vi "add_line_shifted_enface_IMAQ.vi"(0 "En Face Image":T1, 1 "Shift":dbl=1.0, 5 "Raw Image":T1, 7 "Aspect Ratio":dbl=1.0, 9 "Input Line":dbl=1.0, 11 "error in (no error)":errorcluster, 12 "Output Line":i32) -> (4 "En Face Image Out":T1, 15 "error out":errorcluster)   [LabVIEW 2016]
uses:
  <vilib>/vision/Image Controls.llb/IMAQ Image.ctl
  <vilib>/vision/NI_Vision_Development_Module.lvlib
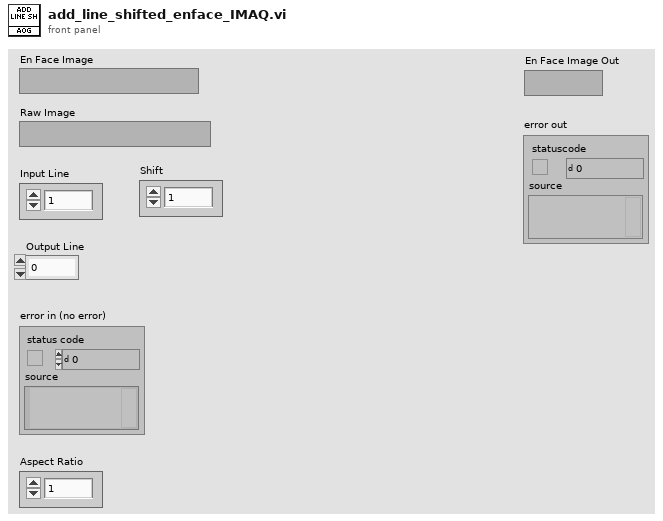
[diagram p1: front panel]
types:
  T1 = typedef "IMAQ Image.ctl" = refnum<image>
  T2 = typedef "Image Type" = u32
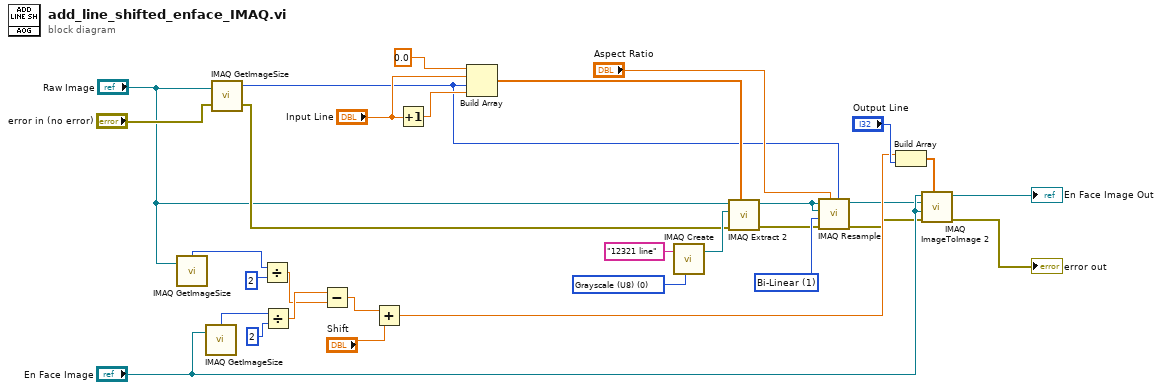
[diagram p0: block diagram]
diagram:
  w6 = u32 1 items=["Zero Order", "Bi-Linear", "Quadratic", "Cubic Spline"] ("Interpolation Type")
  w29 = T2 0 items=["Grayscale (U8)", "Grayscale (I16)", "Grayscale (SGL)", "Complex (CSG)", "RGB (U32)", "HSL (U32)", "RGB (U64)", "Grayscale (U16)"] ("Image Type")
  n1 = call "IMAQ GetImageSize"("Image"="Raw Image") -> ("X Resolution"=w13:i32)  [unwired: 3 in, 2 out]
  n2 = call "IMAQ GetImageSize"("Image"="En Face Image") -> ("X Resolution"=w17:i32)  [unwired: 3 in, 2 out]
  n3 = call "IMAQ GetImageSize"("Image"="Raw Image", "error in (no error)"="error in (no error)") -> ("X Resolution"=w4:i32, "error out"=w21:errorcluster)  [unwired: 2 in, 1 out]
  n4 = Divide(x=w13, y=2) -> (x/y=w11:dbl)
  n5 = Divide(x=w17, y=2) -> (x/y=w12:dbl)
  n6 = Subtract(x=w12, y=w11) -> (x-y=w10:dbl)
  n7 = Add(x=w10, y="Shift") -> (x+y=w8:dbl)
  n8 = Increment(x="Input Line") -> (x+1=w19:dbl)
  n9 = Build Array(0.0 ("element"), "Input Line", w4, w19) -> (w27:dbl[])
  n10 = call "IMAQ Create"("Image Name"="12321 line", "Image Type"=w29) -> ("New Image"=w28:T1)  [unwired: 3 in, 1 out]
  n11 = call "IMAQ Extract 2"("Optional Rectangle"=w27, "error in (no error)"=w21, "Image Dst"=w28, "Image Src"="Raw Image") -> ("error out"=w1:errorcluster, "Image Dst Out"=w7:T1)  [unwired: 6 in]
  n12 = call "IMAQ Resample"("X Resolution"=w4, "Y Resolution"="Aspect Ratio", "error in (no error)"=w1, "Interpolation Type"=w6, "Image Dst"=w7, "Image Src"=w7) -> ("error out"=w2:errorcluster, "Image Dst Out"=w3:T1)  [unwired: 4 in]
  n13 = Build Array(w8, "Output Line") -> (w25:dbl[])
  n14 = call "IMAQ ImageToImage 2"("Offset Left/Top"=w25, "error in (no error)"=w2, "Image Dst"="En Face Image", "Image Src (Small)"=w3, "Image Src (Large)"="En Face Image") -> ("error out"=→"error out":errorcluster, "Image Dst Out"=→"En Face Image Out":T1)  [unwired: 5 in]
